vi "CameraStatusOverTemp.vi"(8 "error in (no error)":errorcluster, 9 "camera":u8, 10 "block":dbl, 11 "sample":dbl) -> (0 "error out":errorcluster, 3 "temp":bool)   [LabVIEW 2015, in "ESLSCDLL.lvlib"]
uses:
  ESLSCDLL.lvlib
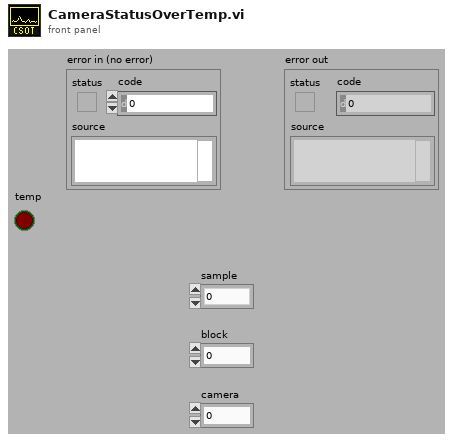
[diagram p1: front panel]
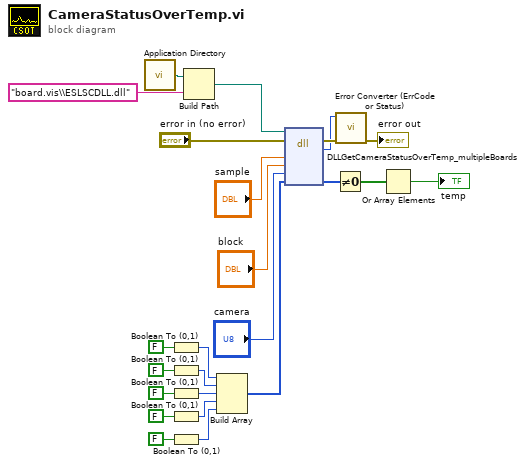
[diagram p0: block diagram]
diagram:
  n1 = call <vilib>:"Application Directory.vi"() -> ("Application Directory"=w20:path)
  n2 = Boolean To (0,1)(Boolean=FALSE) -> (0, 1=w12:i16)
  n3 = Boolean To (0,1)(Boolean=FALSE) -> (0, 1=w11:i16)
  n4 = Boolean To (0,1)(Boolean=FALSE) -> (0, 1=w10:i16)
  n5 = Boolean To (0,1)(Boolean=FALSE) -> (0, 1=w9:i16)
  n6 = Boolean To (0,1)(Boolean=FALSE) -> (0, 1=w8:i16)
  n7 = Build Path(base path=w20, name or relative path="board.vis\\ESLSCDLL.dll") -> (appended path=w18:path)
  n8 = Build Array(w12, w11, w10, w9, w8) -> (w7:i16[])
  n9 = dll-call lib="C:/ENTW/PCIE/LV64/board.vis/ESLSCDLL.dll" fn="DLLGetCameraStatusOverTemp_multipleBoards" ("lwlscdll.dll:DLLWriteLongS0")(path in=w18, error in="error in (no error)", "sample"="sample", "block"="block", "camera_pos"="camera", "tempArr[]"=w7) -> (error out=w22:errorcluster, "es_status_codes"=w21:i32, "tempArr[]"=w3:u8[])  [unwired: 4 in, 1 out]
  n10 = Not Equal To 0?(x=w3) -> (x != 0?=w2:bool[])
  n11 = call "Error Converter (ErrCode or Status).vi"("error in (no error)"=w22, "error code"=w21) -> ("error out"=→"error out":errorcluster)  [unwired: 9 in]
  n12 = Or Array Elements(Boolean array=w2) -> (logical OR=→"temp":bool)
